vi "Write Parameter to Word (U32).vi"(8 "error in":errorcluster, 9 "parameter definition in":T1={"start index"=10, "size"=1, "encoding"=enum."BNR", "signed"=FALSE, "scale multiplier"=1.0, "scale offset"=0.0}, 10 "scaled data":dbl, 11 "32-bit word in":u32 format="%032b") -> (0 "error out":errorcluster, 3 "32-bit word out":u32 format="%032b")   [LabVIEW 2020, in "32-bit Word.lvclass"]
uses:
  ARINC429-32bit/32-bit Word.lvclass
  Parameter Definition.ctl
  <vilib>/NI/NI VeriStand Encoding and Decoding/Encoding.ctl
  ARINC429-32bit/32-bit Word.lvclass/32-bit Word.ctl
  <vilib>/NI/NI VeriStand Encoding and Decoding/Encoding and Decoding.lvlib
  ARINC 429.lvclass
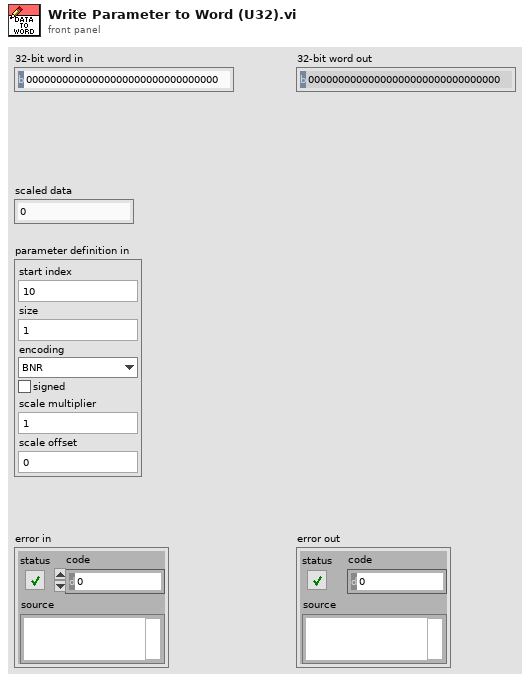
[diagram p1: front panel]
types:
  T1 = typedef "ARINC 429.lvclass/Parameter Definition.ctl" = cluster{"start index":i32, "size":i32, "encoding":T2, "signed":bool, "scale multiplier":dbl, "scale offset":dbl}
  T2 = typedef "Encoding and Decoding.lvlib/Encoding.ctl" = enum16{"BNR", "BCD", "Discrete"}
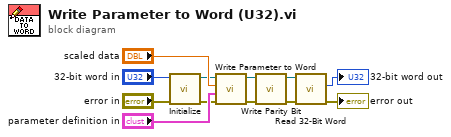
[diagram p0: block diagram]
diagram:
  n1 = call "Initialize.vi"("error in"="error in", "32-bit word"="32-bit word in") -> ("error out"=w1:errorcluster, "ARINC 429 (32-bit word)"=w2:refnum<class "32-bit Word.lvclass">)  [unwired: 8 in]
  n2 = call-dynamic "Write Parameter to Word.vi"("error in"=w1, "parameter definition"="parameter definition in", "data"="scaled data", "32-bit Word in"=w2) -> ("error out"=w4:errorcluster, "32-bit Word out"=w3:refnum<class "32-bit Word.lvclass">)  [unwired: 6 in]
  n3 = call-dynamic "Write Parity Bit.vi"("error in"=w4, "32-bit word in"=w3) -> ("error out"=w5:errorcluster, "32-bit word out"=w6:refnum<class "32-bit Word.lvclass">)  [unwired: 8 in]
  n4 = call "Read 32-Bit Word.vi"("error in (no error)"=w5, "32-bit Word in"=w6) -> ("error out"=→"error out":errorcluster, "32-bit word"=→"32-bit word out":u32)  [unwired: 7 in, 1 out]
